vi "KINECT_Check.vi"(9 "Delta":dbl, 10 "Current":dbl, 11 "Baseline":dbl) -> (3 "In Range?":bool)   [LabVIEW 2011]
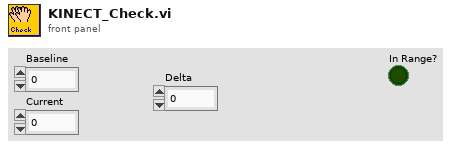
[diagram p1: front panel]
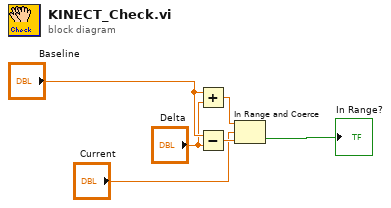
[diagram p0: block diagram]
diagram:
  n1 = Add(x="Baseline", y="Delta") -> (x+y=w4:dbl)
  n2 = Subtract(x="Baseline", y="Delta") -> (x-y=w3:dbl)
  n3 = In Range and Coerce(upper limit=w4, x="Current", lower limit=w3) -> (In Range?=→"In Range?":bool)  [unwired: 1 out]
